vi "ZCAN_GetDeviceInf.vi"(1 "DEVICE_HANDLE":u32, 3 "error in (no error)":errorcluster caption="错误输入（无错误）") -> (5 "DEVICE_HANDLE(out)":u32, 6 "DEVICE_INFO(string out)":string, 8 "error out":errorcluster caption="错误输出")   [LabVIEW 2018]
doc: "该函数用于获取CAN卡（板卡）信息。"
uses:
  data_type/ZCAN_DEVICE_INFO.ctl
panel:
  in  "ZCAN_DEVICE_INFO":T1
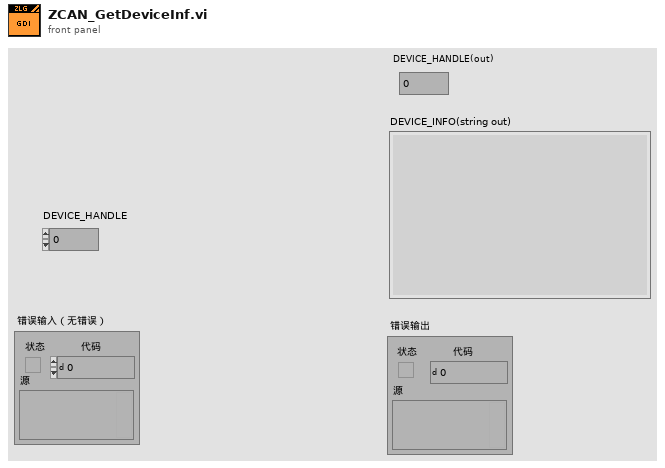
[diagram p1: front panel]
types:
  T1 = typedef "ZCAN_DEVICE_INFO.ctl" = cluster{"hw_Version":u16, "fw_Version":u16, "dr_Version":u16, "in_Version":u16, "irq_Num":u16, "can_Num":u8, "str_Serial_Num":cluster{"str_Serial_Num[0]":u8, "str_Serial_Num[1]":u8, "str_Serial_Num[2]":u8, "str_Serial_Num[3]":u8, "str_Serial_Num[4]":u8, "str_Serial_Num[5]":u8, "str_Serial_Num[6]":u8, "str_Serial_Num[7]":u8, "str_Serial_Num[8]":u8, "str_Serial_Num[9]":u8, "str_Serial_Num[10]":u8, "str_Serial_Num[11]":u8, "str_Serial_Num[12]":u8, "str_Serial_Num[13]":u8, "str_Serial_Num[14]":u8, "str_Serial_Num[15] ":u8, "str_Serial_Num[16] ":u8, "str_Serial_Num[17] ":u8, "str_Serial_Num[18] ":u8, "str_Serial_Num[19]":u8}, "str_hw_Type":cluster{"str_hw_Type[0]":u8, "str_hw_Type[1]":u8, "str_hw_Type[2]":u8, "str_hw_Type[3]":u8, "str_hw_Type[4]":u8, "str_hw_Type[5]":u8, "str_hw_Type[6]":u8, "str_hw_Type[7]":u8, "str_hw_Type[8]":u8, "str_hw_Type[9]":u8, "str_hw_Type[10]":u8, "str_hw_Type[11]":u8, "str_hw_Type[12]":u8, "str_hw_Type[13]":u8, "str_hw_Type[14]":u8, "str_hw_Type[15] ":u8, "str_hw_Type[16] ":u8, "str_hw_Type[17] ":u8, "str_hw_Type[18] ":u8, "str_hw_Type[19]":u8, "str_hw_Type[20]":u8, "str_hw_Type[21]":u8, "str_hw_Type[22]":u8, "str_hw_Type[23]":u8, "str_hw_Type[24]":u8, "str_hw_Type[25]":u8, "str_hw_Type[26]":u8, "str_hw_Type[27]":u8, "str_hw_Type[28]":u8, "str_hw_Type[29]":u8, "str_hw_Type[30]":u8, "str_hw_Type[31]":u8, "str_hw_Type[32]":u8, "str_hw_Type[33]":u8, "str_hw_Type[34]":u8, "str_hw_Type[35] ":u8, "str_hw_Type[36] ":u8, "str_hw_Type[37] ":u8, "str_hw_Type[38] ":u8, "str_hw_Type[39]":u8}, "reserved":cluster{"reserved[0]":u16, "reserved[1] ":u16, "reserved[2] ":u16, "reserved[3] ":u16}}
  T2 = cluster{"str_Serial_Num[0]":u8, "str_Serial_Num[1]":u8, "str_Serial_Num[2]":u8, "str_Serial_Num[3]":u8, "str_Serial_Num[4]":u8, "str_Serial_Num[5]":u8, "str_Serial_Num[6]":u8, "str_Serial_Num[7]":u8, "str_Serial_Num[8]":u8, "str_Serial_Num[9]":u8, "str_Serial_Num[10]":u8, "str_Serial_Num[11]":u8, "str_Serial_Num[12]":u8, "str_Serial_Num[13]":u8, "str_Serial_Num[14]":u8, "str_Serial_Num[15] ":u8, "str_Serial_Num[16] ":u8, "str_Serial_Num[17] ":u8, "str_Serial_Num[18] ":u8, "str_Serial_Num[19]":u8}
  T3 = cluster{"str_hw_Type[0]":u8, "str_hw_Type[1]":u8, "str_hw_Type[2]":u8, "str_hw_Type[3]":u8, "str_hw_Type[4]":u8, "str_hw_Type[5]":u8, "str_hw_Type[6]":u8, "str_hw_Type[7]":u8, "str_hw_Type[8]":u8, "str_hw_Type[9]":u8, "str_hw_Type[10]":u8, "str_hw_Type[11]":u8, "str_hw_Type[12]":u8, "str_hw_Type[13]":u8, "str_hw_Type[14]":u8, "str_hw_Type[15] ":u8, "str_hw_Type[16] ":u8, "str_hw_Type[17] ":u8, "str_hw_Type[18] ":u8, "str_hw_Type[19]":u8, "str_hw_Type[20]":u8, "str_hw_Type[21]":u8, "str_hw_Type[22]":u8, "str_hw_Type[23]":u8, "str_hw_Type[24]":u8, "str_hw_Type[25]":u8, "str_hw_Type[26]":u8, "str_hw_Type[27]":u8, "str_hw_Type[28]":u8, "str_hw_Type[29]":u8, "str_hw_Type[30]":u8, "str_hw_Type[31]":u8, "str_hw_Type[32]":u8, "str_hw_Type[33]":u8, "str_hw_Type[34]":u8, "str_hw_Type[35] ":u8, "str_hw_Type[36] ":u8, "str_hw_Type[37] ":u8, "str_hw_Type[38] ":u8, "str_hw_Type[39]":u8}
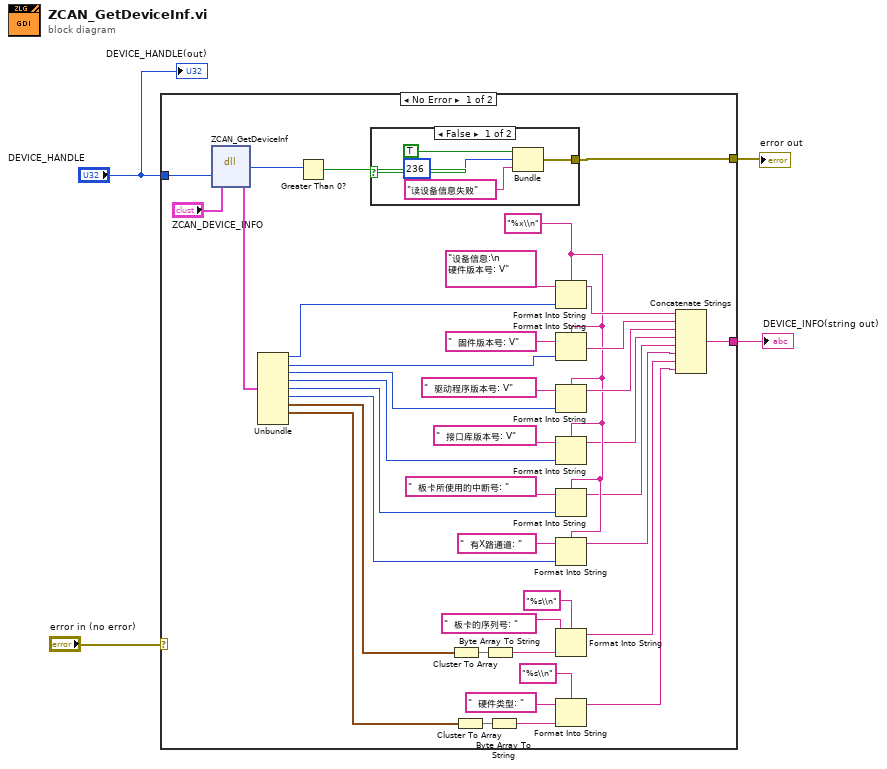
[diagram p0: block diagram]
diagram:
  n1 = case shown="No Error" "error in (no error)" {
    selector: "error in (no error)" -> [_ w47]
    tunnel: [w39 w47] -> w3
    tunnel: "DEVICE_HANDLE" -> [w42 _]
    tunnel: [w9 _] -> w2
    frame No Error {
      w22 = "%x\\n" ("format string")
      n2 = dll-call lib="PTH2qabs CUsersadminDesktopzlgcan_demo_20220516_2018版本zlgcan_demo_USBCANFD_mergebinzlgcan_wrap.dll" fn="ZCAN_GetDeviceInf"("channel_handle"=w42, "ZCAN_DEVICE_INFO") -> ("return"=w41:u32, w37:T1)  [unwired: 4 in, 2 out]
      n3 = Unbundle(w37) -> ("hw_Version"=w5:u16, "fw_Version"=w26:u16, "dr_Version"=w25:u16, "in_Version"=w24:u16, "irq_Num"=w23:u16, "can_Num"=w21:u8, "str_Serial_Num"=w20:T2, "str_hw_Type"=w10:T3)  [unwired: 1 out]
      n4 = Greater Than 0?(x=w41) -> (x > 0?=w40:bool)
      n5 = case shown="False" w40 {
        tunnel: [w43 _] -> w39
        frame False {
          n6 = Bundle("status"=TRUE, "code"=236, "消息"="读设备信息失败") -> (w43:cluster{"status":bool, "code":i32, "消息":string})  [unwired: 1 in]
        }
        frame True {
        }
      }
      n7 = Cluster To Array(cluster=w20) -> (array=w19:u8[])
      n8 = Cluster To Array(cluster=w10) -> (array=w15:u8[])
      n9 = Byte Array To String(unsigned byte array=w19) -> (string=w29:string)
      n10 = Byte Array To String(unsigned byte array=w15) -> (string=w14:string)
      n11 = Format Into String(format string=w22, initial string="设备信息:\n  硬件版本号: V", w5) -> (resulting string=w34:string)  [unwired: 1 in, 1 out]
      n12 = Format Into String(format string=w22, initial string="  固件版本号: V", w26) -> (resulting string=w33:string)  [unwired: 1 in, 1 out]
      n13 = Format Into String(format string=w22, initial string="  驱动程序版本号: V", w25) -> (resulting string=w36:string)  [unwired: 1 in, 1 out]
      n14 = Format Into String(format string=w22, initial string="  接口库版本号: V", w24) -> (resulting string=w18:string)  [unwired: 1 in, 1 out]
      n15 = Format Into String(format string=w22, initial string="  板卡所使用的中断号: ", w23) -> (resulting string=w17:string)  [unwired: 1 in, 1 out]
      n16 = Format Into String(format string=w22, initial string="  有X路通道: ", w21) -> (resulting string=w16:string)  [unwired: 1 in, 1 out]
      n17 = Format Into String(format string="%s\\n", initial string="  板卡的序列号: ", w29) -> (resulting string=w12:string)  [unwired: 1 in, 1 out]
      n18 = Format Into String(format string="%s\\n", initial string="  硬件类型: ", w14) -> (resulting string=w11:string)  [unwired: 1 in, 1 out]
      n19 = Concatenate Strings(w34, w33, w36, w18, w17, w16, w12, w11) -> (w9:string)
    }
    frame Error {
    }
  }
  "error out" <- w3
  "DEVICE_INFO(string out)" <- w2
  "DEVICE_HANDLE(out)" <- "DEVICE_HANDLE"
